vi "UHR-Fleezers Control (host) - 10.5.vi"() -> ()   [LabVIEW 2011] (continued)
  in  "N Acq Sets (Traps + Fl.)":i16=3
  in  "Sets to FIFO (Traps)":T15={"Set 1"=TRUE, "Set 2"=TRUE, "Set 3"=FALSE}
  in  "FPGA Ave.":dbl=1.0 min=1.0 step=1.0
  out "Ave. Period (s)":dbl=5e-06 format="%#_6p"
  out "DMA Update Period (s)":dbl=0.3
  out "FPGA Averaging":bool
  out "Trap Sets":u32=2
  out "Counts/DMA":dbl=12000000.0 format="%#_6p"
  out "Trap Pos FIFO El Remaining":u32=406
  out "Trap Pos Elements/DMA read":u32=120000 format="%.0p"
  out "Trap AI FIFO Timeout":u16
  out "Trap Pos FIFO Timeout":u16
  in  "Video Capture Rate (Hz)":dbl=30.0
  in  "Video Index":dbl=1.0 min=1.0 step=1.0
  in  "New Video File":bool
  in  "Save Video":bool
  in  "Reset Averaging":bool
  in  "Averaging":bool
  in  "Save Image":bool
  in  "Image Index":dbl=1.0 min=1.0
  out "Path Out":path
  in  "Center Point":cluster{"X":i32, "Y":i32}={"X"=335, "Y"=271}
  in  "Zoom Factor":sgl=7.0
  out "Window Size":cluster{"Width":i32, "Height":i32}
  out "Window Position":cluster{"X Position":i32, "Y Position":i32}={"X Position"=40, "Y Position"=40}
  in  "Initial Window Size":cluster{"Width":i32, "Height":i32}={"Width"=884, "Height"=619}
  in  "Initial Window Position":cluster{"X Position":i32, "Y Position":i32}={"X Position"=796, "Y Position"=4}
  in  "Intensity Upper":dbl=88.0
  in  "Intensity Lower":dbl=66.0
  out "error out":errorcluster
  out "error out 2":errorcluster
  in  "Harvard Syringe Pump Serial Port":refnum<visa-resource-name>="ASRL5::INSTR"
  in  "Lost Tether Alarm Threshold (pN)":dbl=0.5
  in  "AOM X Cal (nm/MHz)":dbl=123.0
  in  "MCL X Cal (nm/V)":dbl=1070.0
  out "X RF Amplitude Limits (%)":T16={"Minimum"=0.0, "Maximum"=50.0, "Increment"=1.0}
  out "X RF Frequency Limits (MHz)":T16={"Minimum"=60.0, "Maximum"=90.0, "Increment"=1.0}
  out "Y RF Frequency Limits (MHz)":T16={"Minimum"=0.0, "Maximum"=40.0, "Increment"=1.0}
  out "Y RF Amplitude Limits (%)":T16={"Minimum"=0.0, "Maximum"=50.0, "Increment"=1.0}
  in  "Manip. X?":bool=TRUE
  in  "Manip. Y?":bool
  in  "Force Manip Abort":bool
  out "Read cal error":errorcluster
  in  "DAQ Delay (ms)":u32=1000
  in  "Start Scan":bool
  in  "Scan axis":bool=TRUE
  in  "Osc. amp. (V)":dbl=5.0
  in  "Osc. center (V)":dbl=5.0
  in  "Osc. freq. (Hz) 2":dbl=1.0
  in  "MCL Mode":u16(ring) items=["Manual Positioning", "Sinusoidal Wave", "Linear Scan"]
  in  "Begin (V)":dbl
  in  "End (V)":dbl=10.0
  in  "N Points":dbl=20.0
  in  "Delay to Interlace (s)":dbl
  in  "Delayed Interlace Start":bool
  in  "Read Lateness and Rel Phase":bool
  out "Vec Mean of T1 T2":dbl[](array[numeric])=[-2.4338415969736467, -2.4217851943509956]
  in  "Cal read wait (s)":u32=5
  out "Time tether formed":timestamp=timestamp(3401128904.3086624 s since 1904-01-01)
  in  "Sample Chamber Stage Serial Port":refnum<visa-resource-name>="ASRL4::INSTR"
  in  "Chemyx Syringe Pump Serial Port":refnum<visa-resource-name>="ASRL3::INSTR"
  in  "Limit Min (MHz)":dbl=10.0 caption="Min (MHz)"
  in  "Limit Max (MHz)":dbl=16.0 caption="Max (MHz)"
  in  "Limits Enable":bool=TRUE caption="Enable"
  out "AI labels":string[](array[string])=["T1 Y", "T1 X", "T1 Sum", "T2 Y", "T2 X", "T2 Sum", "T1 FB X", "T1 FB Sum", "T2 FB X", "T2 FB Sum", "PSD Y", "PSD X", "PSD Y Sum"]
  in  "Save Trap Pos. Data":bool=TRUE
  in  "Lower Ch. Cap.":bool
  # "Chemyx Pumps\n(for bead syringes)"
  # "Chemyx Pump 2"
  # "Units: \n1 = ml/m\n2 = ml/h\n3 = ul/m\n4 = ul/h"
  # "Rate param is ul/h\nVolume param is ul"
  # "After"
  # "During"
  # "Trap On?"
  # "BD Flow ON?"
  # "Samp Flow ON?"
  # "Trap Trig. Fl.?"
  # "Zero It"
  # "Floor it\n(e.g., hp unwinding)"
  # "1"
  # "2"
  # "Trap Display:"
  # "APD Display:"
  # "DAQ"
  # "Trap Manipulation"
  # "Data Saving"
  # "Bead Calibration"
  # "Harvard Pump\n(sample channel for flow exp)"
  # "X"
  # "Y"
  # "Oscillate Set 1 freq. (debugging)"
  # "BD 1"
  # "BD 2"
  # "AOD Raster Scan"
  # "Approx. trap separations"
  # "X"
  # "Y"
  # "FPGA\nreading"
  # "DMA\ntransfer"
  # "APD Gates"
  # "APD 2"
  # "APD 1"
  # "X"
  # "2D"
  # "Y"
  # "1D"
  # "Green Laser Interlacing"
  # "Green FB Measurement"
  # "Digital Gate"
  # "Current Analog Control"
  # "Total AI Rates (NOT rates/trap)"
  # "(Samples/trap x Trap Sets)"
  # "(Samples/channel x\n8 if averaging (8 channels)\n4 if no averaging)"
  # "Trap 1"
  # "Trap 2"
  # "Flour./Trap 3"
  # "External Video Window"
  # "MCL Position Debugging"
  # "Temporary Control Storage\n(these used to be somewhere else, still want to keep them)"
  # "Y"
  # "X"
  # "Trap Position Difference Limits"
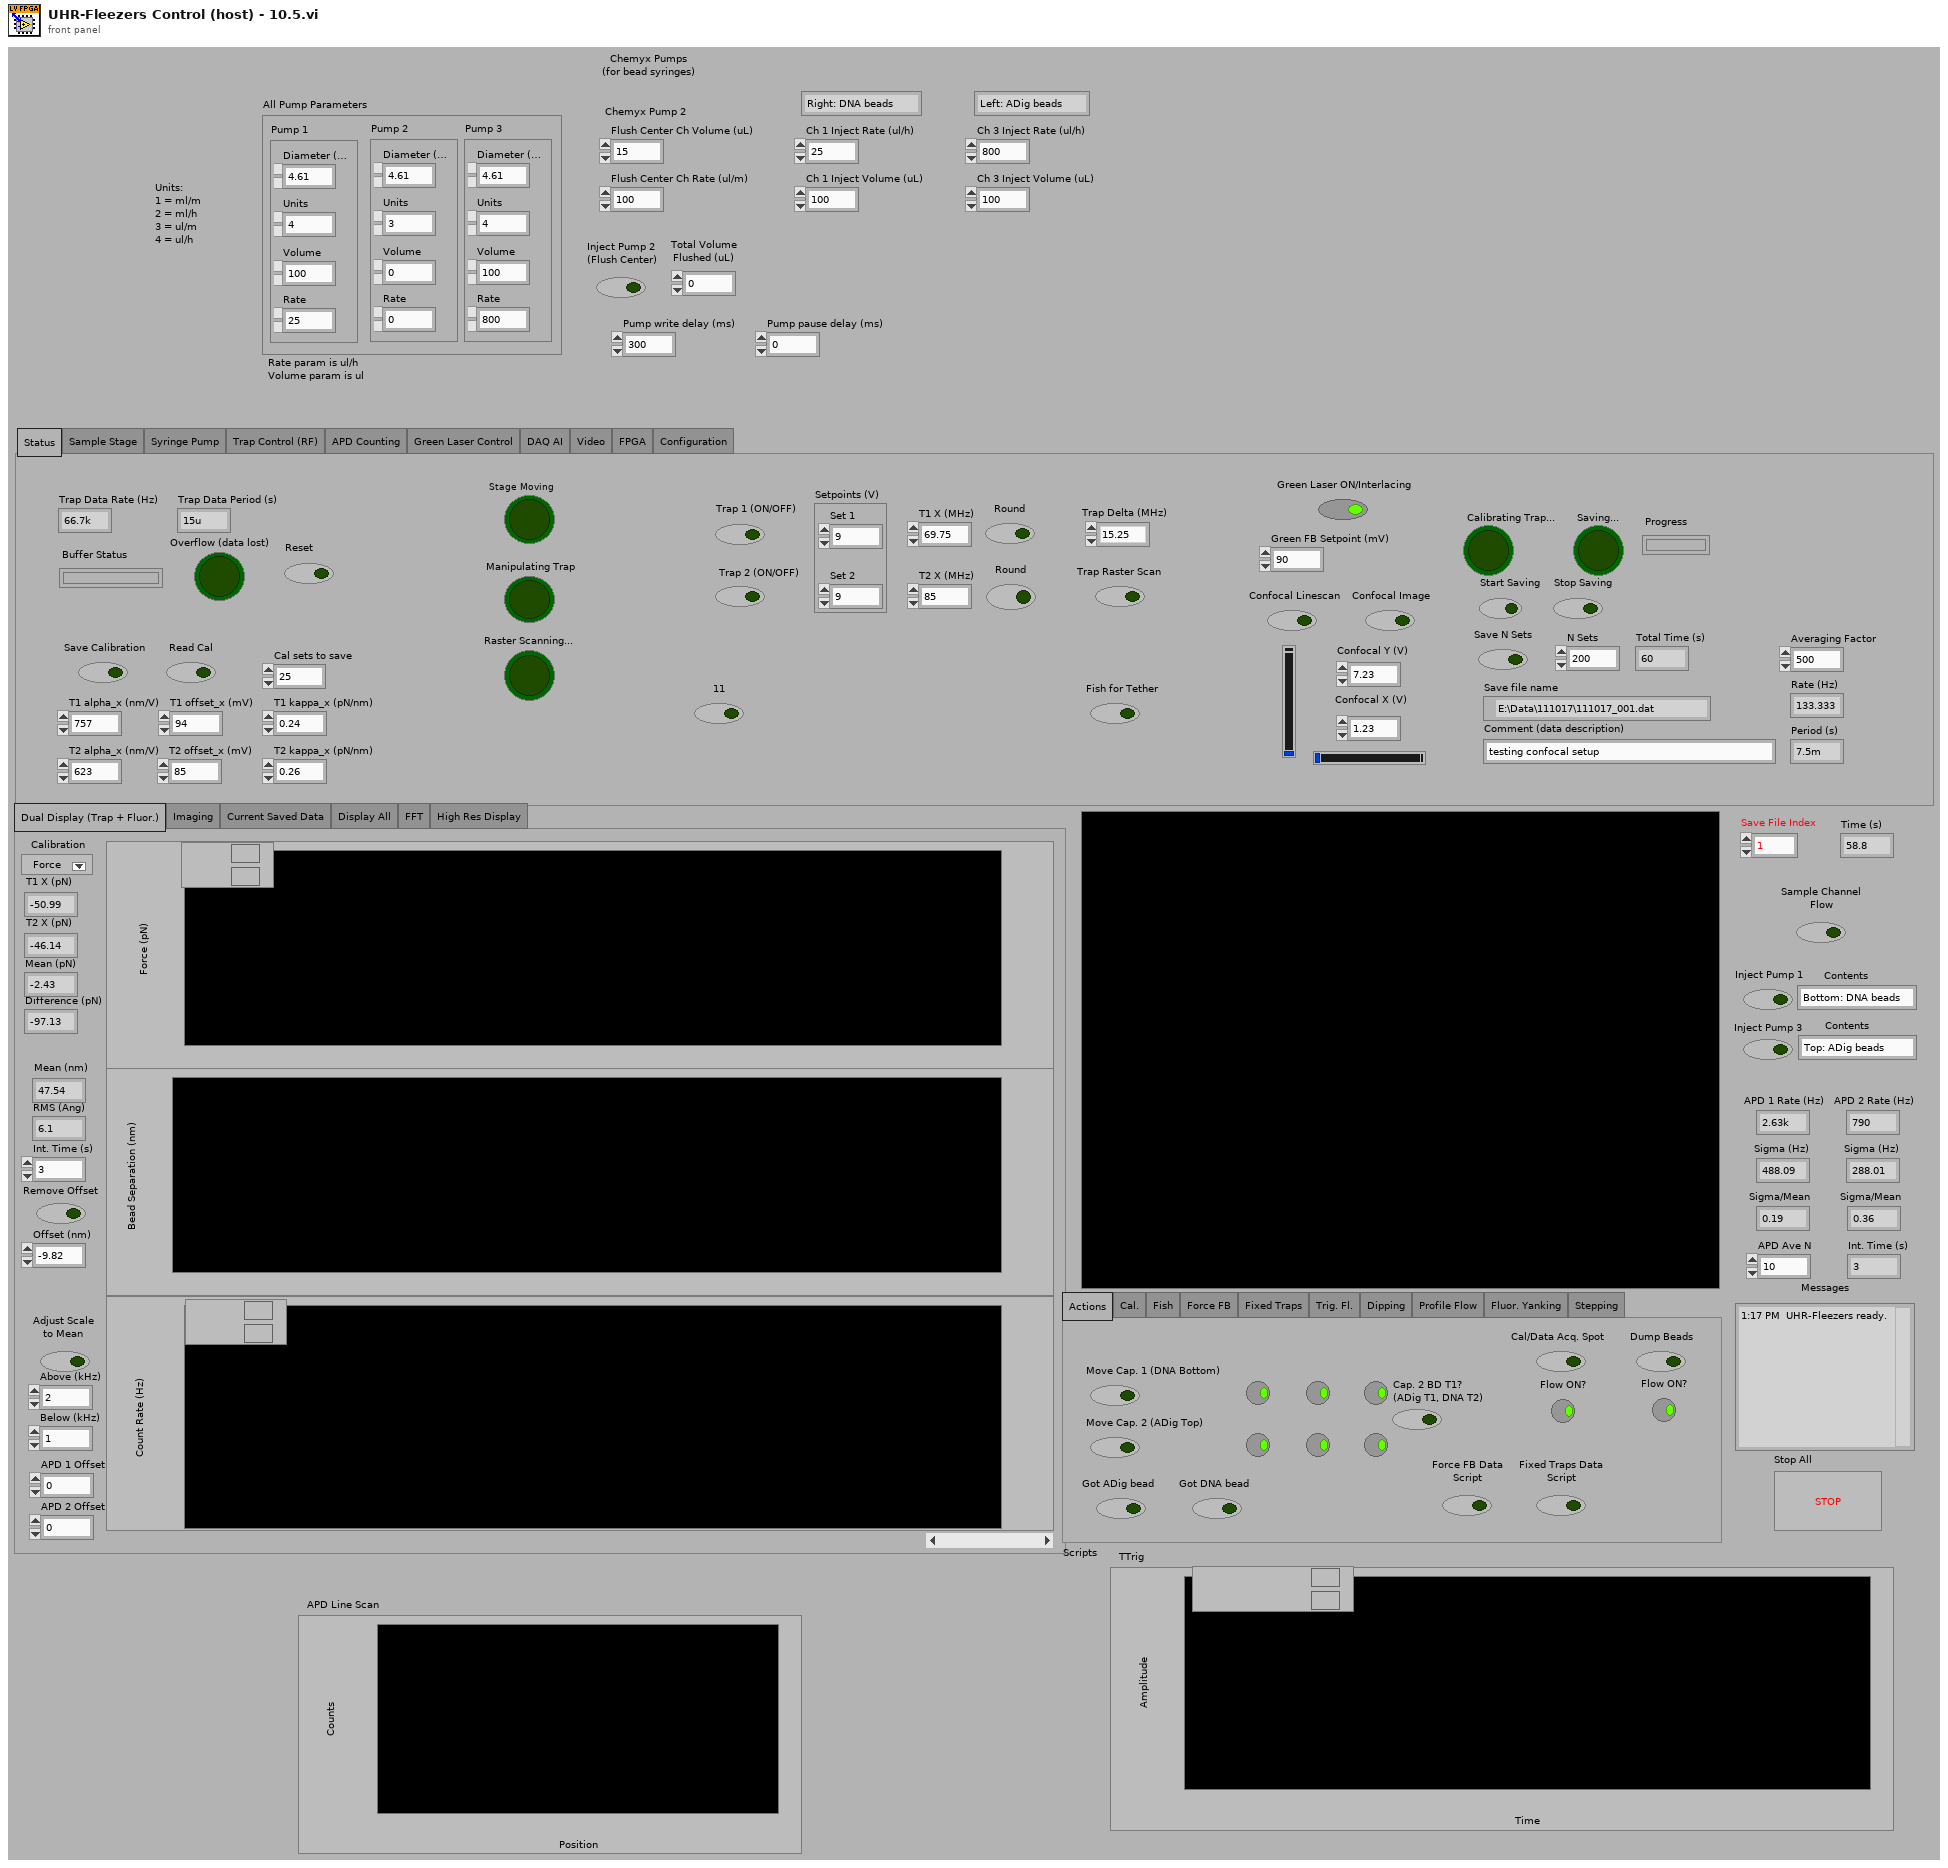
[diagram p1: front panel]
types:
  T1 = cluster{"Pump 1":cluster{"Diameter (mm)":dbl, "Units":dbl, "Volume":dbl, "Rate":dbl}, "Pump 2":cluster{"Diameter (mm)":dbl, "Units":dbl, "Volume":dbl, "Rate":dbl}, "Pump 3":cluster{"Diameter (mm)":dbl, "Units":dbl, "Volume":dbl, "Rate":dbl}}
  T2 = enum32{"Actions", "Cal.", "Fish", "Force FB", "Fixed Traps", "Trig. Fl.", "Dipping", "Profile Flow", "Fluor. Yanking", "Stepping"}
  T3 = typedef "IMAQ Image.ctl" = refnum<image>
  T4 = enum32{"Dual Display (Trap + Fluor.)", "Imaging", "Current Saved Data", "Display All", "FFT", "High Res Display"}
  T5 = enum32{"Status", "Sample Stage", "Syringe Pump", "Trap Control (RF)", "APD Counting", "Green Laser Control", "DAQ AI", "Video", "FPGA", "Configuration"}
  T6 = enum32{"IR Laser Interlacing (Direct RF Board Control Method)", "AOD Raster Scan", "Feedback on Trap Intensity", "Feedback on Trap Position"}
  T7 = typedef "LVPoint32TypeDef.ctl" = cluster{"Horizontal":i32, "Vertical":i32}
  T8 = cluster{"Scan Range AOD (nm) 2":dbl, "Step Size AOD (nm) 2":dbl, "Scan Speed AOD (nm/s) 2":dbl, "Number of scans (AOD) 2":u16, "Label":string}[]
  T9 = cluster{"Set 1":cluster{"proportional gain (Kc)":i16, "integral gain (Kc*Ts/Ti)":i16, "derivative gain (Kc*Td/Ts)":i16}, "Set 2":cluster{"proportional gain (Kc)":i16, "integral gain (Kc*Ts/Ti)":i16, "derivative gain (Kc*Td/Ts)":i16}}
  T10 = cluster{"Trap 1":fxp<+/-,16,1>, "Trap 2":fxp<+/-,16,1>}
  T11 = cluster{"proportional gain (Kc)":fxp<+/-,16,8>, "integral gain (Kc*Ts/Ti)":fxp<+/-,16,8>, "derivative gain (Kc*Td/Ts)":fxp<+/-,16,8>}
  T12 = cluster{"output high":fxp<+/-,16,1>, "output low":fxp<+/-,16,1>}
  T13 = cluster{"Set 1":fxp<+/-,16,1>, "Set 2":fxp<+/-,16,1>}
  T14 = cluster{"proportional gain (Kc)":i16, "integral gain (Kc*Ts/Ti)":i16, "derivative gain (Kc*Td/Ts)":i16}
  T15 = cluster{"Set 1":bool, "Set 2":bool, "Set 3":bool}
  T16 = typedef "LVMinMaxIncTypeDef.ctl" = cluster{"Minimum":dbl, "Maximum":dbl, "Increment":dbl}
  T17 = typedef "Image Type" = u32
  T18 = typedef "nirio_resource_hc.ctl" = tag
  T19 = typedef "openfpgaref.8.6.ctl" = refnum<k20>
  T20 = cluster{"New Image":T3, "New Image":T3, "New Image":T3, "New Image":T3}
  T21 = typedef "XDNodeRunTimeDep.lvlib/timing_clust.ctl" = cluster{"Expected End [f-1]":u64, "Actual End [f-1]":u64, "Finished Late? [f-1]":bool, "Expected End [i-1]":u64, "Actual End [i-1]":u64, "Finished Late? [i-1]":bool, "Expected Start [i]":u64, "Actual Start [i]":u64, "Expected Start [f]":u64, "Actual Start [f]":u64, "Source Name":string, "Structure Name":string, "Period":i64, "Deadline":i64, "Offset":i64, "Start":i64, "Priority":i32, "Timeout":i32, "Mode":T22, "Wakeup Reason":T23, "Error":errorcluster, "Source Type":string, "Secondary Source Type":string, "Global End Time":u64, "Global Start Time":u64, "Frame Duration":u64, "Iteration Duration":u64, "Assigned CPU":i32, "I/O Scan Engine Mode":u32}
  T22 = typedef "XDNodeRunTimeDep.lvlib/nitl_modes.ctl" = enum32{"No Change", "Process missed periods, maintain original phase", "Discard missed periods, maintain original phase", "Process missed periods, ignore original phase", "Discard missed periods, ignore original phase"}
  T23 = typedef "XDNodeRunTimeDep.lvlib/wakeup.ctl" = enum32{"Normal", "Aborted", "Asynchronous wakeup", "Timing source error", "Timed loop error", "Timeout"}
  T24 = enum16{"big-endian, network order", "native, host order", "little-endian"}
  T25 = enum16{"open", "replace", "create", "open or create", "replace or create", "replace or create with confirmation"}
  T26 = cluster{"Scan Range AOD (nm) 2":dbl, "Step Size AOD (nm) 2":dbl, "Scan Speed AOD (nm/s) 2":dbl, "Number of scans (AOD) 2":u16, "Label":string}
  T27 = cluster{"[0]":dbl, "[1]":dbl, "[2]":dbl, "[3]":dbl, "[4]":dbl, "[5]":dbl}
  T28 = cluster{"Diameter (mm)":dbl, "Units":dbl, "Volume":dbl, "Rate":dbl}
  T29 = cluster{"Left":i32, "Top":i32, "Width":u32, "Height":u32}
  T30 = cluster{cluster{"Left":i32, "Top":i32, "Width":u32, "Height":u32}}[]
  T31 = enum32{"setting", "request", "request control", "info", "statistics", "system settings", "I/O sub system", "HRT control", "camera descriptions", "device specific data", "event sub system settings", "event sub system results", "image memory manager"}
  T32 = typedef "AviRefnum.ctl" = refnum<k1>
  T33 = typedef "imagedata.ctl" = cluster{"image type":i32, "image depth":i32, "image":u8[], "mask":u8[], "colors":u32[], "Rectangle":cluster{"left":i16, "top":i16, "right":i16, "bottom":i16}}
  T34 = enum32{"Normal Display", "Dual Display (APD)", "FFT", "High Res Display"}
  T35 = cluster{"Origin Pixel":cluster{"X":sgl, "Y":sgl}, "Angle Relative to Horizontal (deg)":sgl, "Axis Reference":u32}
  T36 = typedef "Simple Grid Descriptor" = cluster{"X Step":sgl, "Y Step":sgl, "Unit":T37}
  T37 = typedef "Image Unit" = enum32{"Undefined", "Angström", "Micrometer", "Millimeter", "Centimeter", "Meter", "Kilometer", "Microinch", "Inch", "Feet", "Nautical miles", "Standard miles", "Steps"}
  T38 = cluster{"averaging mode":u16, "weighting mode":u16, "number of averages":u32}
  T39 = cluster{"dB On (F)":bool, "unwrap phase (F)":bool, "convert to degree (F)":bool}
  T40 = cluster{string, string, string, string, string, string, string, string}
  T41 = cluster{string, string, string, string, string, string, string, string, string, string, string, string}
  T42 = cluster{string, string, string, string, string, string, string, string, string, string, string, string, string}
  T43 = cluster{string, string, string, string, string, string, string, string, string, string, string, string, string, string}
  T44 = cluster{"BD 1 Frequency 1 (MHz)":dbl, "BD 1 Frequency 2 (MHz)":dbl}
  T45 = cluster{"f0":dbl, "df":dbl, "magnitude":dbl[]}[][]
  T46 = cluster{"Green FB Ch 0":i16, "Green FB Ch 1":i16, "Green FB Ch 2":i16}
  T47 = cluster{"Green FB Ch 0":dbl, "Green FB Ch 1":dbl, "Green FB Ch 2":dbl}
diagram:
  w57 = u16 20 items=["1.0"=10, "1.5"=15, "2.0"=20] ("stop bits (10: 1 bit)")
  w64 = T17 2 items=["Grayscale (U8)", "Grayscale (I16)", "Grayscale (SGL)", "Complex (CSG)", "RGB (U32)", "HSL (U32)", "RGB (U64)", "Grayscale (U16)"] ("Image Type")
  w127 = cluster{"output high":i16, "output low":i16} {"output high"=3000, "output low"=0} ("FB output range 1")
  w198 = 10.0 ("y")
  w197 = 32767.0 ("y")
  w213 = 6.0  # clock mult.
  w214 = 49152000.0  # TCXO frequ.
  n1 = Build Array("DIO count 1 (ticks)", "DIO count 2 (ticks)", "DIO count 3 (ticks)") -> (w114:u32[])
  n2 = local read "AO1"() -> (w192:dbl)
  n3 = local read "AO2"() -> (w191:dbl)
  n4 = local read "Scan Increment (MHz)"() -> (w209:dbl)
  n5 = local read "Continuous MCL Scanning"() -> (w179:bool)
  n6 = local read "Fast Scan Dir"() -> (w178:bool)
  n7 = local read "Number of scans (MCL)"() -> (w180:u64)
  n8 = property on="AI Count (ticks)" class="DigNum (strict)"("Val(Sgnl)"="AI Count (ticks)") -> ()  [unwired: 2 in, 2 out]
  n9 = Multiply(x=w192, y=w197) -> (x*y=w194:dbl)
  n10 = Multiply(x=w191, y=w197) -> (x*y=w196:dbl)
  n11 = Divide(x=w194, y=w198) -> (x/y=w193:dbl)
  n12 = Divide(x=w196, y=w198) -> (x/y=w195:dbl)
  n13 = To Word Integer(number=w193) -> (16bit integer=w190:i16)
  n14 = To Word Integer(number=w195) -> (16bit integer=w189:i16)
  n15 = Not(x=w178) -> (.not. x?=w173:bool)
  n16 = local read "Cycles/step (MCL)"() -> (w181:u64)
  n17 = Multiply(x=w209, y=1000.0) -> (x*y=w216:dbl)
  n18 = local read "Scan steps (MCL)"() -> (w182:u64)
  n19 = local write "Trap Pos FIFO Timeout"(u16 0 ("Trap Pos FIFO Timeout")) -> ()
  n20 = local read "Desired Scan Incr (V)"() -> (w184:dbl)
  n21 = Scale By Power Of 2(n=48, x=w216) -> (x*2^n=w217:dbl)
  n22 = Multiply(x=w214, y=w213) -> (x*y=w212:dbl)
  n23 = Divide(x=w217, y=w212) -> (x/y=w211:dbl)
  n24 = local read "Setpoints (V)"() -> (w230:cluster{"Set 1":dbl, "Set 2":dbl})
  n25 = To Quad Integer(1:w211) -> (0:w208:i64)
  n26 = Divide(x=40000000.0, y="AI Count (ticks)") -> (x/y=w169:dbl)
  n27 = Multiply(x=w184, y=32767.0) -> (x*y=w186:dbl)
  n28 = local read "Number Interlace Sets"() -> (w107:u8)
  n29 = Split 1D Array(array=w114, index=w107) -> (first subarray=w116:u32[])  [unwired: 1 out]
  n30 = Add Array Elements(numeric array=w116) -> (sum=w115:u32)
  n31 = local read "# Samples/channel"() -> (w201:u32)
  n32 = local read "Number of F/B Scans (AOD)"() -> (w202:u16)
  n33 = local read "Not-Interlacing Set"() -> (w106:enum32{"Set 1", "Set 2", "Set 3"})
  n34 = To Unsigned Byte Integer(number=w106) -> (unsigned 8bit integer=w112:u8)
  n35 = Index Array(array=w114, index=w112) -> (element=w113:u32)
  n36 = local read "Feedback On/Off"() -> (w233:cluster{"Set 1":bool, "Set 2":bool})
  n37 = local read "PID Gains"() -> (w225:T9)
  n38 = local read "Scan steps (AOD)"() -> (w207:u64)
  n39 = local read "All FB On/Off"() -> (w234:bool)
  n40 = local read "Cycles/step (AOD)"() -> (w206:u64)
  n41 = local write "AI rate (Hz)"(w169) -> ()
  n42 = Divide(x=w186, y=10.0) -> (x/y=w185:dbl)
  n43 = Multiply(x=w207, y=w206) -> (x*y=w205:u64)
  n44 = Multiply(x=3276.7, y=w230) -> (x*y=w229:cluster{"Set 1":dbl, "Set 2":dbl})
  n45 = xnode "FPGA Open VI Reference"("resource name"=T18 "750kHzDAQ") -> ("FPGA VI Reference Out"=w222:T19, "error out"=w221:errorcluster)  [unwired: 1 in]
  n46 = To Word Integer(number=w185) -> (16bit integer=w183:i16)
  n47 = Multiply(x=w205, y=u64 2) -> (x*y=w203:u64)
  n48 = local read "Sets to FIFO (Traps)"() -> (w237:T15)
  n49 = Divide(x=w169, y="FPGA Ave.") -> (x/y=w170:dbl)
  n50 = To Word Integer(number=w229) -> (16bit integer=w228:cluster{"Set 1":i16, "Set 2":i16})
  n51 = Unbundle By Name(w225) -> ("Set 1"=w224:T14, "Set 2"=w223:T14)
  n52 = Multiply(x=w203, y=w202) -> (x*y=w200:u64)
  n53 = local write "Ave. Rate (Hz)"(w170) -> ()
  n54 = Divide(x=w200, y=w201) -> (x/y=w199:dbl)
  n55 = Unbundle By Name(w228) -> ("Set 1"=w227:i16, "Set 2"=w226:i16)
  n56 = local read "2D or 1D Scan"() -> (w128:bool)
  n57 = local write "Data points/scans"(w200) -> ()
  n58 = local read "Scan BD"() -> (w218:bool)
  n59 = And(x=w233, y=w234) -> (x .and. y?=w232:cluster{"Set 1":bool, "Set 2":bool})
  n60 = local write "Data points/scan (f/b)"(w203) -> ()
  n61 = Reciprocal(x=w170) -> (1/x=w171:dbl)
  n62 = local read "N Acq Sets (Traps + Fl.)"() -> (w162:i16)
  n63 = local write "N sets should be saved"(w199) -> ()
  n64 = xnode "Invoke Method"("FPGA VI Reference In"=w222, "error in"=w221) -> ("FPGA VI Reference Out"=w126:T19, "error out"=w136:errorcluster)
  n65 = Unbundle By Name(w232) -> ("Set 1"=w236:bool, "Set 2"=w235:bool)
  n66 = local read "Interlace"() -> (w108:bool)
  n67 = Select(t=w115, s=w108, f=w113) -> (s? t:f=w105:u32)
  n68 = local write "Update Count (MCL)"(w105) -> ()
  n69 = local write "Total Counts (ticks)"(w105) -> ()
  n70 = local write "Ave. Period (s)"(w171) -> ()
  n71 = property on="2D or 1D Scan" class="Bool (strict)"("Val(Sgnl)"=w128) -> ()  [unwired: 2 in, 2 out]
  n72 = local read "GI Frequency, OFF count"() -> (w28:u32)
  n73 = local read "GI Frequency, ON count"() -> (w19:u32)
  n74 = local read "APD Gate OFF Count"() -> (w25:u32)
  n75 = local read "APD Gate ON Count"() -> (w21:u32)
  n76 = xnode "Read/Write Control"("FPGA VI Reference In"=w125, "error in"=w136, "ai count"="AI Count (ticks)", "Interlace ON/OFF"=w108, "Number Interlace Cycles"=w107, "AI1 Sets to FIFO"=w237, "FB On/Off Set 1"=w236, "FB On/Off Set 2"=w235, "Interlace Off Parameters"=w106, "FB Setpoint Set 1"=w227, "FB Setpoint Set 2"=w226, "FB Gains Set 1"=w224, "FB Gains Set 2"=w223, "FB output range 1"=w127, "FB output range 2"=w127, "Cycles per step"=w206, "Scan BD"=w218, "Number of scans"=w202, "Scan steps"=w207, "Scan freq.  increment"=w208, "AO1"=w190, "AO2"=w189, "Scan freq.  increment (MCL)"=w183, "Scan steps (MCL)"=w182, "Cycles per step (MCL)"=w181, "Number of scans (MCL)"=w180, "MCL count"=w105, "Cont. Scan (MCL)"=w179, "MCL Scan Axis"=w173, "1D or 2D Scan?"=w128, "N of AI1 Int Acq Sets"=w162, "Freq or Amp switch first"="Freq or Amp switch first", "Freq switch delay"="Freq switch delay", "Amp switch delay"="Amp switch delay", "Swap F1 and F2"="Swap F1 and F2", "APD to FIFO"=FALSE, "DIO count 1 (ticks)"="DIO count 1 (ticks)", "DIO count 2 (ticks)"="DIO count 2 (ticks)", "DIO count 3 (ticks)"="DIO count 3 (ticks)") -> ("FPGA VI Reference Out"=w32:T19, "error out"=w30:errorcluster)  [unwired: 1 in]
  n77 = local read "On one out of X cycles"() -> (w27:u32)
  n78 = local read "APD Integration Time (s)"() -> (w11:dbl)
  n79 = local read "DMA Update Period (s)"() -> (w10:dbl)
  n80 = Add(x=w21, y=w25) -> (x+y=w23:u32)
  n81 = Add(x=w19, y=w28) -> (x+y=w26:u32)
  n82 = local read "Green Laser ON/Interlacing"() -> (w103:bool)
  n83 = local read "Green laser mode"() -> (w104:enum32{"Laser ON", "Laser OFF", "Interlace"})
  n84 = Multiply(x=w23, y=w27) -> (x*y=w24:u32)
  n85 = Multiply(x=w27, y=w26) -> (x*y=w18:u32)
  n86 = Reciprocal(x=w11) -> (1/x=w8:dbl)
  n87 = Multiply(x=w11, y=40000000.0) -> (x*y=w7:dbl)
  n88 = Divide(x=w10, y=w11) -> (x/y=w13:dbl)
  n89 = Multiply(x="Current When FB OFF (%)", y=655.35) -> (x*y=w91:dbl)
  n90 = local read "Invert APD Gate"() -> (w17:bool)
  n91 = Multiply(x="Green FB Setpoint (mV)", y=3.2767) -> (x*y=w88:dbl)
  n92 = local read "APD Gate"() -> (w16:enum32{"ON", "OFF", "Interlace"})
  n93 = Subtract(x=w24, y=w21) -> (x-y=w22:u32)
  n94 = local write "Green FB Count"(w18) -> ()
  n95 = local write "APD Acq Rate (Hz)"(w8) -> ()
  n96 = To Unsigned Long Integer(number=w7) -> (unsigned 32bit integer=w5:u32)
  n97 = Multiply(x=2.0, y=w13) -> (x*y=w12:dbl)
  n98 = local read "Invert GI"() -> (w100:bool)
  n99 = To Unsigned Word Integer(number=w91) -> (unsigned 16bit integer=w89:u16)
  n100 = Subtract(x=w18, y=w19) -> (x-y=w20:u32)
  n101 = local write "APD Samples/FIFO Acq."(w13) -> ()
  n102 = To Word Integer(number=w88) -> (16bit integer=w86:i16)
  n103 = local write "APD Elements/DMA read"(w12) -> ()
  n104 = case shown="False" w103 {
    tunnel: w104 -> [_ w263]
    tunnel: [enum32{"Laser ON", "Laser OFF", "Interlace"}."Laser OFF" ("Green laser mode") w263] -> w99
    frame False {
    }
    frame True {
    }
  }
  n105 = local write "APD Int. Count"(w5) -> ()
  n106 = local read "Trap Pos. AI1 X Pre-scale"() -> (w43:u16)
  n107 = local read "Trap Pos FB Monitor\nT1 or T2"() -> (w50:bool)
  n108 = local read "Trap Pos FB Int Count"() -> (w36:u16)
  n109 = local read "APD 1 AO Mult."() -> (w15:i16)
  n110 = local read "Trap Pos FB Negate Action"() -> (w49:bool)
  n111 = local read "APD 2 AO Mult."() -> (w14:i16)
  n112 = local read "Trap Pos. FB Offset Factor"() -> (w48:i64)
  n113 = local read "Trap Pos. FB Mult Factor"() -> (w47:i64)
  n114 = local read "Differential FB?"() -> (w2:bool)
  n115 = local read "Neg. TTrig FPGA"() -> (w4:bool)
  n116 = local read "Trap Pos. FB Gains"() -> (w45:T11)
  n117 = local read "Trap Pos. FB Range"() -> (w46:T12)
  n118 = xnode "Read/Write Control"("FPGA VI Reference In"=w32, "error in"=w30, "Invert APD Gate"=w17, "APD Gate ON Count"=w21, "APD Gate OFF Count"=w22, "APD Acq Rate Count"=w5, "APD Gate Operating Mode"=w16, "APD 1 AO scale factor"=w15, "APD 2 AO scale factor"=w14, "Green interlace ON count"=w19, "Green interlace OFF count"=w20, "Green interlace ON count 2"=w19, "Green interlace OFF count 2"=w20, "Green FB Count"=w18) -> ("FPGA VI Reference Out"=w31:T19, "error out"=w29:errorcluster)
  n119 = xnode "Read/Write Control"("FPGA VI Reference In"=w31, "error in"=w29, "Invert GI 2"=w100, "Operating Mode 2"=w99, "Green FB Gains"="Green FB Gains", "Green FB Setpoint"=w86, "Green FB On/Off"="Green FB On/Off", "Current Out"=w89, "Green int current ON count adj"="Green int current ON count adj", "Operating Mode"=w99, "Invert GI"=w100, "Trap Pos FB Monitor T1 or T2"=w50, "Trap Pos FB Negate Action"=w49, "Trap Pos. FB Offset Factor"=w48, "Trap Pos. FB Mult Factor"=w47, "Trap Pos. FB Range"=w46, "Trap Pos. FB Gains"=w45, "Force feedback"=FALSE, "AI1 X Scale"=w43, "Trap Pos to FIFO"=TRUE, "Trap Pos FB Int Count"=w36, "TTrig Negate Pos"=w4, "FB Trig Integrate"="FB Trig Integrate", "Diff FB Measurement?"=w2, "Negate Diff?"="Negate Diff?") -> ("FPGA VI Reference Out"=w101:T19, "error out"=w102:errorcluster)
  n120 = xnode "Invoke Method"("FPGA VI Reference In"=w101, "error in"=w102, "Depth"="Trap AI FIFO Depth") -> ("FPGA VI Reference Out"=w53:T19, "error out"=w52:errorcluster)
  n121 = xnode "Invoke Method"("FPGA VI Reference In"=w53, "error in"=w52, "Depth"="Trap Position FIFO Depth") -> ("FPGA VI Reference Out"=w38:T19, "error out"=w37:errorcluster)
  n122 = flat-sequence {
    tunnel: w126 -> [w268]
    tunnel: [w268] -> w125
    tunnel: [w267] -> w124
    tunnel: [w266] -> w123
    tunnel: [w264] -> w121
    tunnel: [w265] -> w122
    frame #0 {
      w265 = T16 {"Minimum"=0.0, "Maximum"=40.0, "Increment"=1.0} ("Min Max Inc")
      w264 = T16 {"Minimum"=0.0, "Maximum"=50.0, "Increment"=1.0} ("Data Entry Limits")
      w267 = T16 {"Minimum"=60.0, "Maximum"=90.0, "Increment"=1.0} ("Min Max Inc")
      w266 = T16 {"Minimum"=0.0, "Maximum"=50.0, "Increment"=1.0} ("Data Entry Limits")
      n123 = property on="BD 2 Frequency 1 (MHz)" class="DigNum (strict)"("Data Range"=w265) -> ()  [unwired: 2 in, 2 out]
      n124 = property on="BD 2 Frequency 3 (MHz)" class="DigNum (strict)"("Data Range"=w265) -> ()  [unwired: 2 in, 2 out]
      n125 = property on="BD 2 Frequency 2 (MHz)" class="DigNum (strict)"("Data Range"=w265) -> ()  [unwired: 2 in, 2 out]
      n126 = property on="BD 1 Frequency 1 (MHz)" class="DigNum (strict)"("Data Range"=w267) -> ()  [unwired: 2 in, 2 out]
      n127 = property on="BD 1 Frequency 2 (MHz)" class="DigNum (strict)"("Data Range"=w267) -> ()  [unwired: 2 in, 2 out]
      n128 = property on="BD 1 Frequency 3 (MHz)" class="DigNum (strict)"("Data Range"=w267) -> ()  [unwired: 2 in, 2 out]
      n129 = property on="BD 2 Amplitude 1 (%)" class="DigNum (strict)"("Data Range"=w264) -> ()  [unwired: 2 in, 2 out]
      n130 = property on="BD 2 Amplitude 2 (%)" class="DigNum (strict)"("Data Range"=w264) -> ()  [unwired: 2 in, 2 out]
      n131 = property on="BD 2 Amplitude 3 (%)" class="DigNum (strict)"("Data Range"=w264) -> ()  [unwired: 2 in, 2 out]
      n132 = property on="BD 1 Amplitude 3 (%)" class="DigNum (strict)"("Data Range"=w266) -> ()  [unwired: 2 in, 2 out]
      n133 = property on="BD 1 Amplitude 2 (%)" class="DigNum (strict)"("Data Range"=w266) -> ()  [unwired: 2 in, 2 out]
      n134 = property on="BD 1 Amplitude 1 (%)" class="DigNum (strict)"("Data Range"=w266) -> ()  [unwired: 2 in, 2 out]
      "X RF Frequency Limits (MHz)" <- w267
      "X RF Amplitude Limits (%)" <- w266
      "Y RF Amplitude Limits (%)" <- w264
      "Y RF Frequency Limits (MHz)" <- w265
    }
  }
  n135 = xnode "Invoke Method"("FPGA VI Reference In"=w38, "error in"=w37) -> ("FPGA VI Reference Out"=w135:T19, "error out"=w134:errorcluster)  [unwired: 1 in]
  n136 = flat-sequence "Initial FPGA Loop Relative Phase Adjustment" {
    tunnel: "Initial Phase Adjustment (AI1)" -> [w279]
    tunnel: "Initial Phase Adjustment (GI)" -> [w278]
    tunnel: w135 -> [w277]
    tunnel: w134 -> [w276]
    tunnel: "Initial Phase Adj. (MCL)" -> [w275]
    tunnel: [w280] -> w144
    tunnel: [w274] -> w140
    tunnel: "Initial Phase Adjustment (APD Acq)" -> [w273]
    tunnel: "Initial Phase Adjustment (APD 1 Gate)" -> [w272]
    tunnel: "Initial Phase Adjustment (Green FB)" -> [w271]
    tunnel: "Initial Phase Adjustment (GI) 2" -> [w270]
    tunnel: "Initial Phase Adjustment (APD 2 Gate)" -> [w269]
    tunnel: w144 -> [w282]
    tunnel: [w283] -> w141
    tunnel: w140 -> [w283]
    tunnel: [w282] -> w139
    tunnel: w141 -> [w286]
    tunnel: w139 -> [w285]
    tunnel: [w288] -> w138
    tunnel: [w287] -> w137
    tunnel: [w290] -> w142
    tunnel: [w291] -> w143
    tunnel: w138 -> [w291]
    tunnel: w137 -> [w290]
    frame #0 {
      n137 = xnode "Read/Write Control"("FPGA VI Reference In"=w277, "error in"=w276, "Phase count adjustment"=w279, "Phase count adjustment (GI)"=w278, "Phase count adjustment (MCL)"=w275, "Phase Count Adjustment (APD Acq)"=w273, "Phase count adjustment (APD 1 Gate)"=w272, "Phase count adjustment (APD 2 Gate)"=w269, "Phase count adjustment (Green FB)"=w271, "Phase count adjustment (GI) 2"=w270) -> ("FPGA VI Reference Out"=w274:T19, "error out"=w280:errorcluster)
    }
    frame #1 {
      n138 = Wait (ms)(milliseconds to wait=u32 100) -> ()  [unwired: 1 out]
    }
    frame #2 {
      w284 = TRUE
